vi "User_Event_LV2.vi"(0 "STOP":T1, 11 "Error In":errorcluster, 13 "Operation":T2) -> (4 "User Event Ref":refnum<user-event>, 15 "Error Out":errorcluster)   [LabVIEW 2020, in "Data Communication Transmitter.lvlib"]
doc: "User Event LV2. Used to stop the producer loop when the consumer halts."
uses:
  Data Communication Transmitter.lvlib
  Typedefs/User_Event_Operation.ctl
  Typedefs/User_Event_STOP.ctl
panel:
  # "USER EVENT LV2"
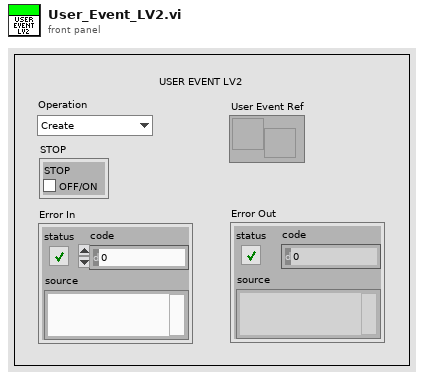
[diagram p1: front panel]
types:
  T1 = typedef "Data Communication Transmitter.lvlib/User_Event_STOP.ctl" = cluster{"STOP":bool}
  T2 = typedef "Data Communication Transmitter.lvlib/User_Event_Operation.ctl" = enum16{"Create", "Generate", "Destroy", "Get Ref"}
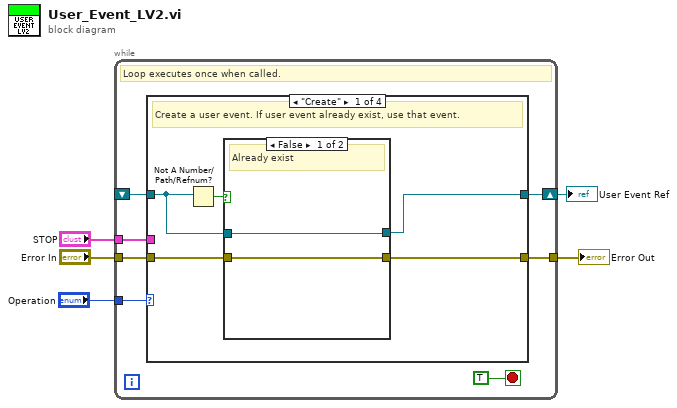
[diagram p0: block diagram]
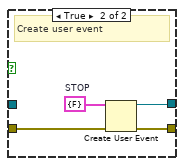
[diagram p2: hidden frame]
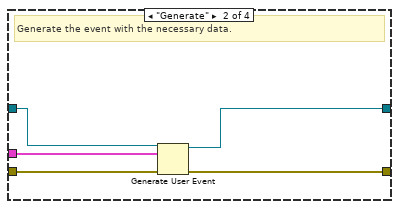
[diagram p3: hidden frame]
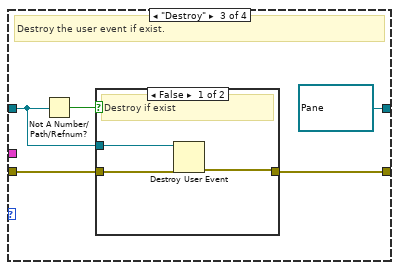
[diagram p4: hidden frame]
diagram:
  n1 = while {
    tunnel: "Operation" -> [w12]
    shift-right: [w11] -> w1
    shift-left: _ -> [w10]
    tunnel: "Error In" -> [w9]
    tunnel: [w8] -> w3
    tunnel: "STOP" -> [w6]
    stop <- TRUE stop-if-true
    # "Loop executes once when called."
    n2 = case shown="\"Create\"" w12 {
      tunnel: [w13 w25 refnum<user-event> refnum ("Datatype") w39] -> w11
      tunnel: w10 -> [w14 w26 w30 w39]
      tunnel: w9 -> [w16 w28 w32 w38]
      tunnel: [w15 w27 w31 w38] -> w8
      tunnel: w6 -> [_ w24 _ _]
      frame "Create" {
        # "Create a user event. If user event already exist, use that event."
        n3 = Not A Number/Path/Refnum?(number/path/refnum=w14) -> (NaN/Path/Refnum?=w17:bool)
        n4 = case shown="False" w17 {
          tunnel: [w19 w23] -> w13
          tunnel: w16 -> [w18 w22]
          tunnel: [w18 w21] -> w15
          tunnel: w14 -> [w19 _]
          frame False {
            # "Already exist"
          }
          frame True {
            w20 = cluster{"STOP":bool} {"STOP"=FALSE}  # STOP
            # "Create user event"
            n5 = Create User Event(user event datatype=w20, error in=w22) -> (user event=w23:refnum<user-event>, error out=w21:errorcluster)
          }
        }
      }
      frame "Generate" {
        # "Generate the event with the necessary data."
        n6 = Generate User Event(user event=w26, event data cluster=w24, error in=w28) -> (user event out=w25:refnum<user-event>, error out=w27:errorcluster)  [unwired: 1 in]
      }
      frame "Destroy" {
        # "Destroy the user event if exist."
        n7 = Not A Number/Path/Refnum?(number/path/refnum=w30) -> (NaN/Path/Refnum?=w33:bool)
        n8 = case shown="False" w33 {
          tunnel: w32 -> [w36 w37]
          tunnel: [w35 w37] -> w31
          tunnel: w30 -> [w34 _]
          frame False {
            # "Destroy if exist"
            n9 = Destroy User Event(user event=w34, error in=w36) -> (error out=w35:errorcluster)
          }
          frame True {
            # "User Event doesnot exist"
          }
        }
      }
      frame "Get Ref" {
        # "Get the User Event Reference"
      }
    }
  }
  "Error Out" <- w3
  "User Event Ref" <- w1
